vi "remove unwanted characters from string.vi"(9 "replace with (_)":string="_", 10 "unwanted patterns/characters":string[](array[string]), 11 "string in":string) -> (3 "string out":string)   [LabVIEW 2013, in "Shared Memory editor node.lvclass"]
uses:
  Shared Memory editor node.lvclass
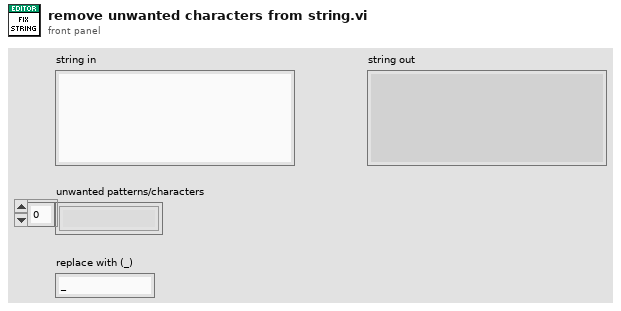
[diagram p1: front panel]
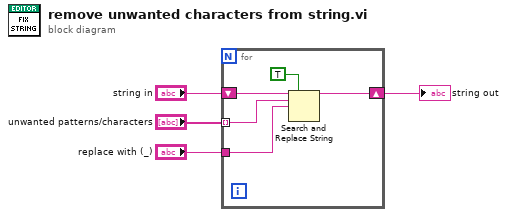
[diagram p0: block diagram]
diagram:
  n1 = for {
    shift-right: [w8] -> w1
    shift-left: "string in" -> [w9]
    tunnel: "unwanted patterns/characters" -> [w7] mode=indexing
    tunnel: "replace with (_)" -> [w6]
    n2 = Search and Replace String(replace all?=TRUE ("replace all? (F)"), input string=w9, search string=w7, replace string=w6) -> (result string=w8:string)  [unwired: 4 in, 3 out]
  }
  "string out" <- w1
